vi "Line Sensor position SubVI.vi"(0 "Array":dbl[](array[numeric]), 1 "error in (no error)":errorcluster) -> (2 "Sensor Values\n(Mapped)":cluster{"Z1":dbl, "Z2":dbl, "Z3":dbl, "Z4":dbl}, 3 "Position":dbl, 4 "Raw sensor values":T2, 5 "error out":errorcluster)   [LabVIEW 2018]
uses:
  <vilib>/myRIO/Common/Instrument Driver Framework/myRIO v1.0/AI/typedefs/AI Channels List.ctl
  <vilib>/myRIO/Common/Instrument Driver Framework/myRIO v1.0/AI/typedefs/AI Channels Enum.ctl
panel:
  out "Black":T1
  out "Mapped S4":dbl
  out "Mapped S3":dbl
  out "Mapped S2":dbl
  out "Mapped S1":dbl
  out "S4 voltage":dbl
  out "S3 voltage":dbl
  out "S2 Voltage":dbl
  out "S1 voltage":dbl
  in  "stop":bool
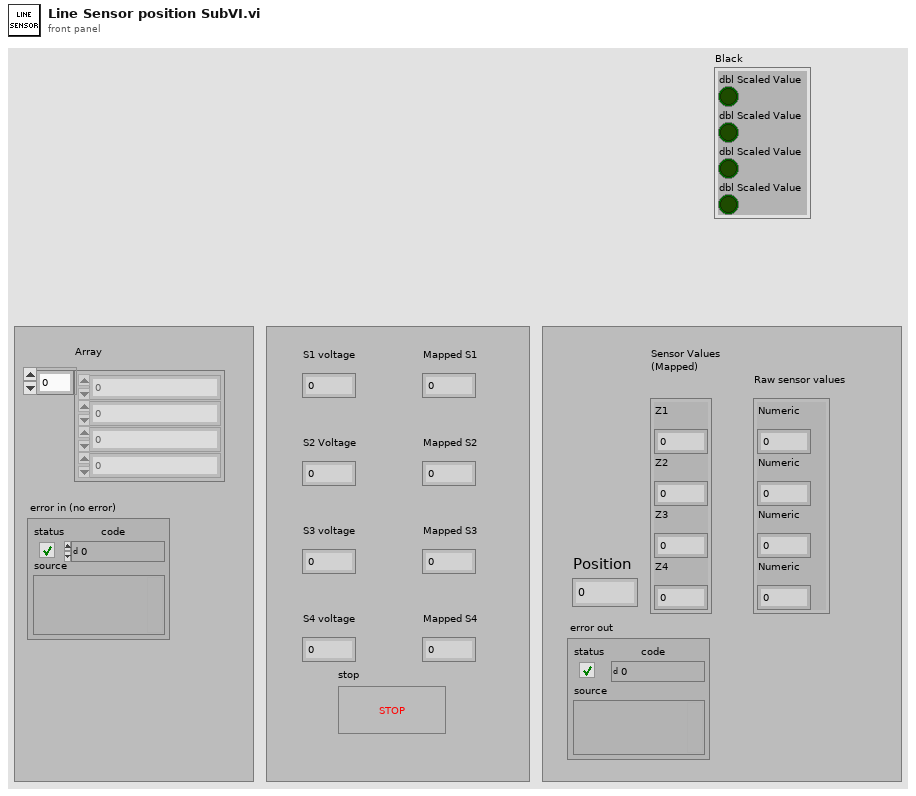
[diagram p1: front panel]
types:
  T1 = cluster{"dbl Scaled Value":bool, "dbl Scaled Value":bool, "dbl Scaled Value":bool, "dbl Scaled Value":bool}
  T2 = cluster{"Numeric":dbl, "Numeric":dbl, "Numeric":dbl, "Numeric":dbl}
  T3 = typedef "AI Channels List.ctl" = T4[]
  T4 = typedef "AI Channels Enum.ctl" = enum16{"Not Connected", "AudioIn/Left", "AudioIn/Right", "C/AI0", "C/AI1", "A/AI0", "A/AI1", "A/AI2", "A/AI3", "A/AI4", "A/AI5", "A/AI6", "A/AI7", "B/AI0", "B/AI1", "B/AI2", "B/AI3", "B/AI4", "B/AI5", "B/AI6", "B/AI7", "AI/AI0", "AI/AI1", "AI/AI2", "AI/AI3", "A/AI0 (DIFF)", "A/AI1 (DIFF)", "A/AI2 (DIFF)", "A/AI3 (DIFF)", "B/AI0 (DIFF)", "B/AI1 (DIFF)", "B/AI2 (DIFF)", "B/AI3 (DIFF)"}
  T5 = typedef "Analog Scaling Constants List.ctl" = T6[]
  T6 = typedef "Analog Scaling Constants.ctl" = cluster{"LSB Weight (Volts)":dbl, "Offset (Volts)":dbl, "Signed?":bool}
  T7 = cluster{"Scale Constants Array":T5, "FPGA Reference Out":refnum<k20>, "AI Channel":T3}
  T8 = cluster{"dbl Scaled Value":dbl, "dbl Scaled Value":dbl, "dbl Scaled Value":dbl, "dbl Scaled Value":dbl}
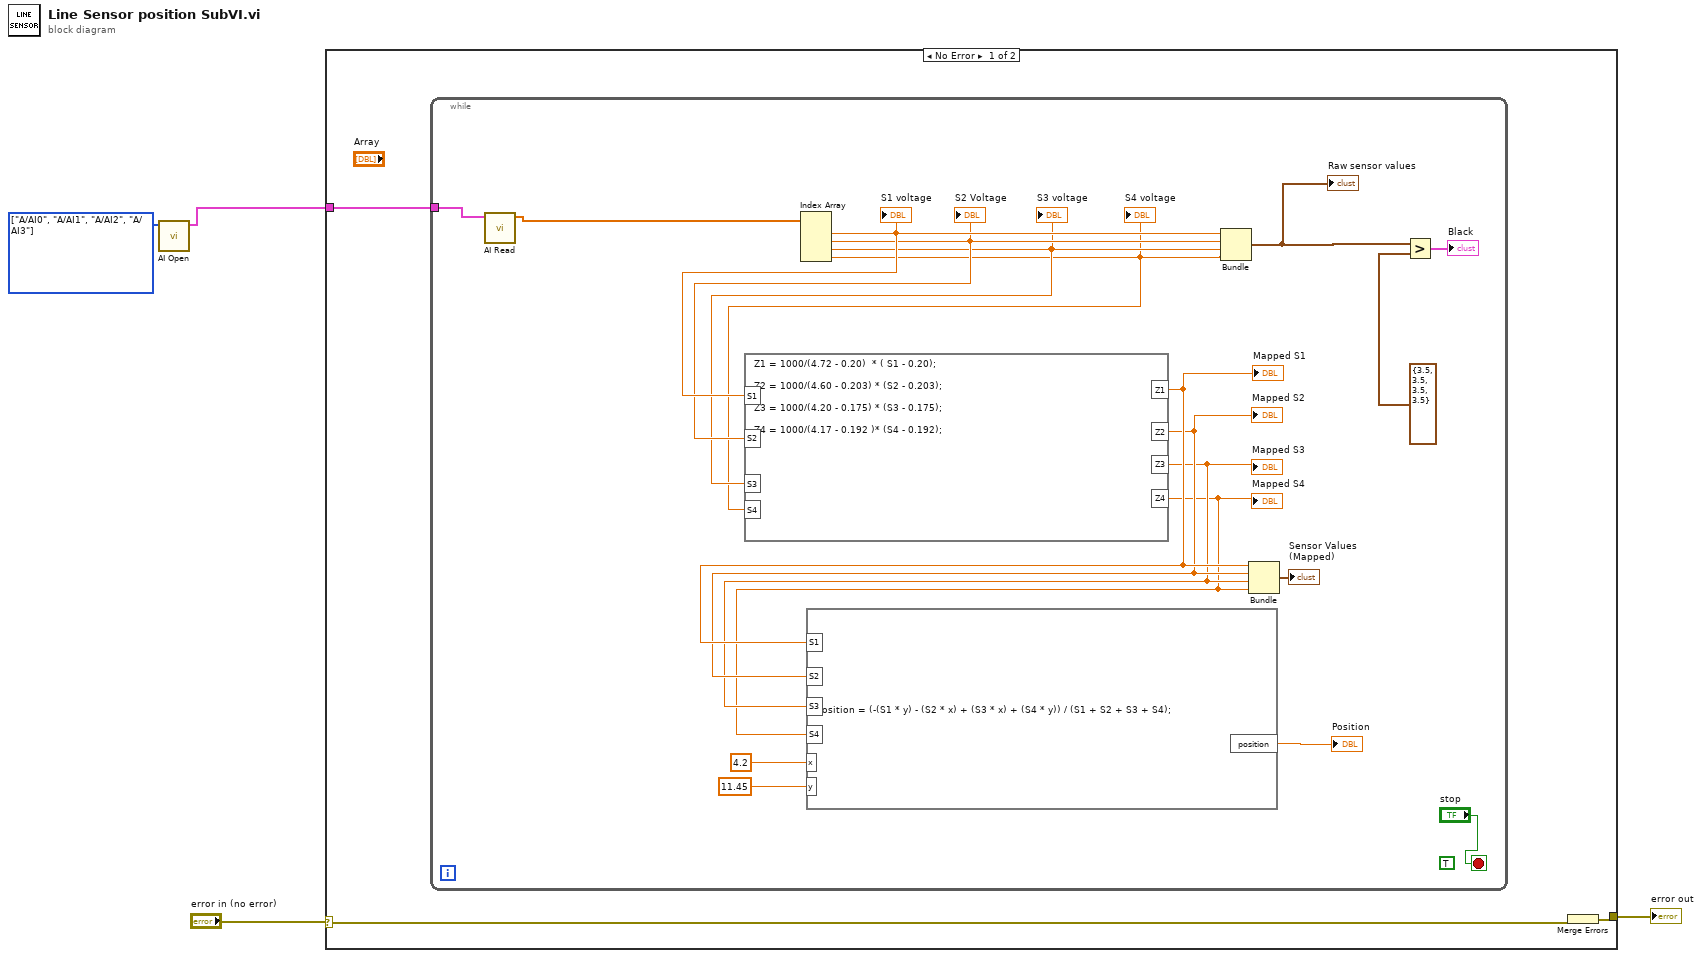
[diagram p0: block diagram]
diagram:
  w2 = T3 [enum."A/AI0", enum."A/AI1", enum."A/AI2", enum."A/AI3"] items=["Not Connected", "AudioIn/Left", "AudioIn/Right", "C/AI0", "C/AI1", "A/AI0", "A/AI1", "A/AI2", "A/AI3", "A/AI4", "A/AI5", "A/AI6", "A/AI7", "B/AI0", "B/AI1", "B/AI2", "B/AI3", "B/AI4", "B/AI5", "B/AI6", "B/AI7", "AI/AI0", "AI/AI1", "AI/AI2", "AI/AI3", "A/AI0 (DIFF)", "A/AI1 (DIFF)", "A/AI2 (DIFF)", "A/AI3 (DIFF)", "B/AI0 (DIFF)", "B/AI1 (DIFF)", "B/AI2 (DIFF)", "B/AI3 (DIFF)"] ("AI Channel")
  n1 = call <vilib>:"AI Open.vi"("AI Channel"=w2) -> ("Analog Info"=w1:T7)  [unwired: 9 in, 1 out]
  n2 = case shown="No Error" "error in (no error)" {
    selector: "error in (no error)" -> [w6 w26]
    tunnel: [w7 w26] -> w3
    tunnel: w1 -> [w5 _]
    frame No Error {
      n3 = while {
        tunnel: w5 -> [w12]
        stop <- "stop" stop-if-true
        (unwired) TRUE
        n4 = call <vilib>:"AI Read.vi"("Analog Info"=w12) -> ("Array"=w11:dbl[])  [unwired: 9 in, 1 out]
        n5 = Index Array(array=w11) -> (element #1=w17:dbl, element #2=w16:dbl, element #3=w15:dbl, element #4=w14:dbl)  [unwired: 4 in]
        "S1 voltage" <- w17
        "S2 Voltage" <- w16
        "S3 voltage" <- w15
        "S4 voltage" <- w14
        n6 = formula code="Z1 = 1000/(4.72 - 0.20)  * ( S1 - 0.20);\n\nZ2 = 1000/(4.60 - 0.203) * (S2 - 0.203);\n\nZ3 = 1000/(4.20 - 0.175) * (S3 - 0.175);\n\nZ4 = 1000/(4.17 - 0.192 )* (S4 - 0.192);"("S1"=w17, "S2"=w16, "S3"=w15, "S4"=w14) -> ("Z1"=w22:dbl, "Z2"=w21:dbl, "Z3"=w20:dbl, "Z4"=w19:dbl)
        "Mapped S1" <- w22
        "Mapped S2" <- w21
        "Mapped S3" <- w20
        "Mapped S4" <- w19
        n7 = formula code="position = (-(S1 * y) - (S2 * x) + (S3 * x) + (S4 * y)) / (S1 + S2 + S3 + S4);"("S1"=w22, "S2"=w21, "S3"=w20, "S4"=w19, "x"=4.2 ("input variable"), "y"=11.45 ("input variable")) -> ("position"=→"Position":dbl)
        n8 = Bundle("dbl Scaled Value"=w17, "dbl Scaled Value"=w16, "dbl Scaled Value"=w15, "dbl Scaled Value"=w14) -> (w10:T8)  [unwired: 1 in]
        "Raw sensor values" <- w10
        n9 = Bundle("Z1"=w22, "Z2"=w21, "Z3"=w20, "Z4"=w19) -> (→"Sensor Values\n(Mapped)":cluster{"Z1":dbl, "Z2":dbl, "Z3":dbl, "Z4":dbl})  [unwired: 1 in]
        n10 = Greater?(x=w10, y=T8 {"dbl Scaled Value"=3.5, "dbl Scaled Value"=3.5, "dbl Scaled Value"=3.5, "dbl Scaled Value"=3.5}) -> (0:→"Black":T1)
      }
      n11 = Merge Errors(w6) -> (w7:errorcluster)
    }
    frame Error {
    }
  }
  "error out" <- w3
